vi "letterToNumber.vi"(1 "letter":string) -> (0 "number":u8)   [LabVIEW 2015]
doc: "returns the corresponding number of <b>letter</b>: A=1, Z=26.\nUpper and lower case letters are accepted.\nNon-letter characters return 0.\nOnly the first character or <b>letter</b> string is read."
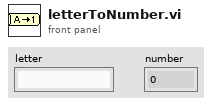
[diagram p1: front panel]
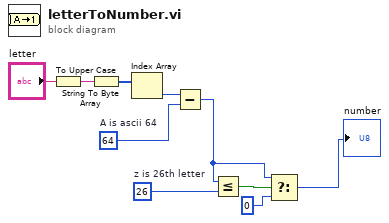
[diagram p0: block diagram]
diagram:
  w5 = u8 26  # z is 26th letter
  w6 = u8 64  # A is ascii 64
  n1 = To Upper Case(1:"letter") -> (0:w10:string)
  n2 = String To Byte Array(string=w10) -> (unsigned byte array=w7:u8[])
  n3 = Index Array(array=w7) -> (element=w8:u8)  [unwired: 1 in]
  n4 = Subtract(x=w8, y=w6) -> (x-y=w3:u8)
  n5 = Less Or Equal?(x=w3, y=w5) -> (x <= y?=w4:bool)
  n6 = Select(t=w3, s=w4, f=u8 0) -> (s? t:f=→"number":u8)
